vi "Core_[TCPIP]Not Connect.vi"(8 "error in (no error)":errorcluster, 11 "HSMS Class in":refnum<class "HSMS Class.lvclass">) -> (0 "error out":errorcluster, 3 "HSMS Class out":refnum<class "HSMS Class.lvclass">)   [LabVIEW 2020, in "SECS Communication.lvlib" / "HSMS Class.lvclass"]
uses:
  HSMS Class.lvclass
  HSMS State.ctl
  Notifier Type.ctl
  HSMS Class.lvclass/HSMS Class.ctl
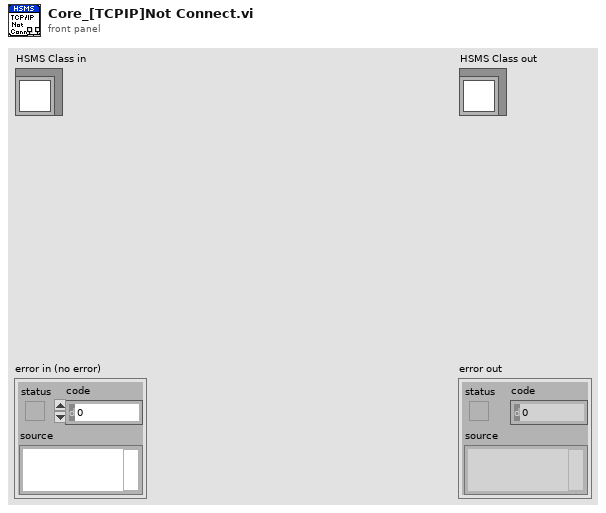
[diagram p1: front panel]
types:
  T1 = typedef "SECS Communication.lvlib/HSMS Class.lvclass/Notifier Type.ctl" = enum16{"TCPIP Connect", "TCPIP Disconnect", "Receive Message", "Send Message", "T3 Timeout", "T6 Timeout", "T7 Timeout", "Error", "Stop"}
  T2 = typedef "SECS Communication.lvlib/HSMS Class.lvclass/HSMS State.ctl" = enum16{"[TCP/IP]Not Connect", "[HSMS]Not Selected", "[HSMS]Selected", "Stop"}
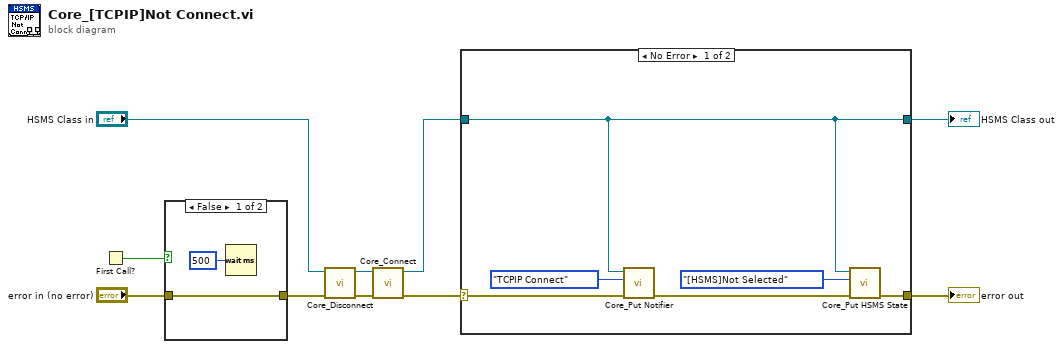
[diagram p0: block diagram]
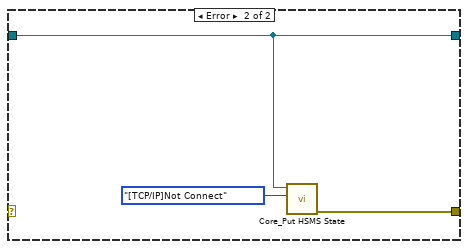
[diagram p3: hidden frame]
diagram:
  n1 = First Call?() -> (First Call?: T/F=w7:bool)
  n2 = case shown="False" w7 {
    tunnel: [w11 w13] -> w4
    tunnel: "error in (no error)" -> [w11 w13]
    frame False {
      n3 = Wait (ms)(milliseconds to wait=u32 500) -> ()  [unwired: 1 out]
    }
    frame True {
    }
  }
  n4 = call "Core_Disconnect.vi"("error in (no error)"=w4, "HSMS Class in"="HSMS Class in") -> ("error out"=w3:errorcluster, "HSMS Class out"=w2:refnum<class "HSMS Class.lvclass">)  [unwired: 8 in]
  n5 = call "Core_Connect.vi"("error in (no error)"=w3, "HSMS Class in"=w2) -> ("error out"=w5:errorcluster, "HSMS Class out"=w6:refnum<class "HSMS Class.lvclass">)  [unwired: 8 in]
  n6 = case shown="No Error" w5 {
    selector: w5 -> [w16 _]
    tunnel: w6 -> [w14 w21]
    tunnel: [w14 w21] -> w10
    tunnel: [w19 w20] -> w9
    frame No Error {
      n7 = call "Core_Put Notifier.vi"("error in (no error)"=w16, "Notifier Type"=Notifier_Type."TCPIP Connect", "HSMS Class in"=w14) -> ("error out"=w15:errorcluster)  [unwired: 7 in, 1 out]
      n8 = call "Core_Put HSMS State.vi"("error in (no error)"=w15, "HSMS State"=HSMS_State."[HSMS]Not Selected", "HSMS Class in"=w14) -> ("error out"=w19:errorcluster)  [unwired: 7 in, 1 out]
    }
    frame Error {
      n9 = call "Core_Put HSMS State.vi"("HSMS State"=HSMS_State."[TCP/IP]Not Connect", "HSMS Class in"=w21) -> ("error out"=w20:errorcluster)  [unwired: 8 in, 1 out]
    }
  }
  "error out" <- w9
  "HSMS Class out" <- w10
